vi "Configure Multi Eval Meas Trigger.vi"(0 "VISA resource name":refnum<visa-resource-name>, 1 "Trigger Threshold (-20.0)":dbl=-20.0 format="%^.3e", 2 "Minimum Trigger Gap (500e-6)":dbl=0.0005 format="%^.3e", 5 "Instance (1)":T1=1, 7 "Trigger Source (\"IF Power\")":string="IF Power", 9 "Trigger Slope (Rising)":i32(ring) items=["Rising", "Falling"], 11 "error in (no error)":errorcluster, 12 "Trigger Delay (0)":dbl format="%^.3e", 13 "Sync Mode (Normal)":i32(ring) items=["Normal", "Enhanced"]) -> (4 "VISA resource name out":refnum<visa-resource-name>, 15 "error out":errorcluster)   [LabVIEW 2020, in "Rohde&Schwarz CMWXP NR FR1 Measurement.lvlib"]
doc: "Configures multi evaluation measurement trigger subsystem.\n\nAttributes:\nRSCMWXPNRFR1M_ATTR_MULTI_EVAL_MEAS_TRIGGER_SOURCE\nRSCMWXPNRFR1M_ATTR_MULTI_EVAL_MEAS_TRIGGER_SLOPE\nRSCMWXPNRFR1M_ATTR_MULTI_EVAL_MEAS_TRIGGER_THRESHOLD\nRSCMWXPNRFR1M_ATTR_MULTI_EVAL_MEAS_TRIGGER_DELAY\nRSCMWXPNRFR1M_ATTR_MULTI_EVAL_MEAS_MINIMUM_TRIGGER_GAP\nRSCMWXPNRFR1M_ATTR_MULTI_EVAL_MEAS_TRIGGER_SYNC_MODE\n\nRemote-control commands:\nTRIGger:NRSub:MEAS<i>:MEValuation:SOURce\nTRIGger:NRSub:MEAS<i>:MEValuation:SLOPe\nTRIGger:NRSub:MEAS<i>:MEValuation:THReshold\nTRIGger:NRSub:MEAS<i>:MEValuation:DELay\nTRIGger:NRSub:MEAS<i>:MEValuation:MGAP\nTRIGger:NRSub:MEAS<i>:MEValuation:SMODe"
uses:
  <instrlib>/Rohde&Schwarz CMWXP NR FR1 Measurement/Rohde&Schwarz CMWXP NR FR1 Measurement.lvlib
  <instrlib>/Rohde&Schwarz CMWXP NR FR1 Measurement/Private/_Instance.ctl
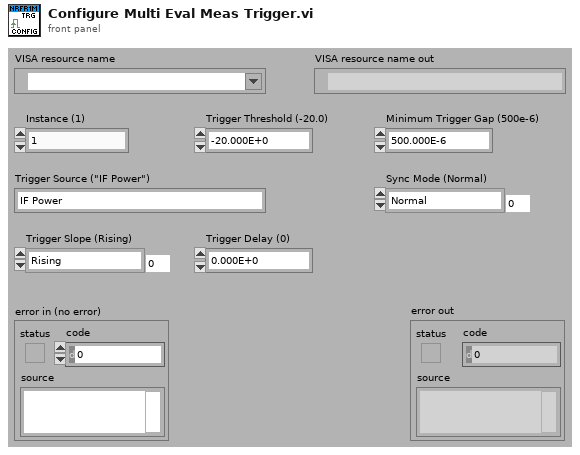
[diagram p1: front panel]
types:
  T1 = typedef "Rohde&Schwarz CMWXP NR FR1 Measurement.lvlib/_Instance.ctl" = i32
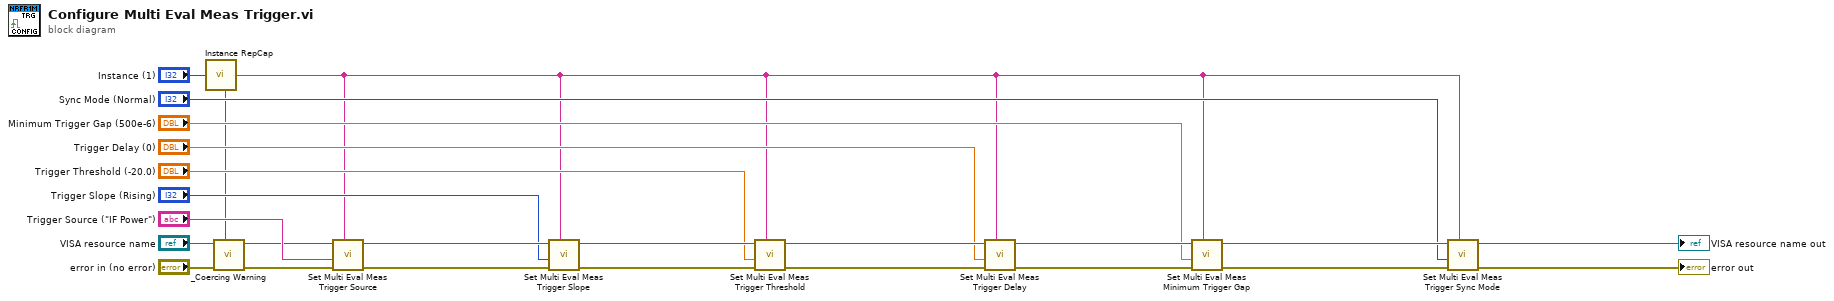
[diagram p0: block diagram]
diagram:
  n1 = call <instrlib>:"Instance RepCap.vi"("Instance In"="Instance (1)") -> ("In Range?"=w1:bool, "RepCap Identifier Out"=w6:string)  [unwired: 1 in]
  n2 = call <instrlib>:"_Coercing Warning.vi"("In Range?"=w1, "error in (no error)"="error in (no error)", "VISA resource name"="VISA resource name") -> ("error out"=w3:errorcluster, "VISA resource name out"=w2:refnum<visa-resource-name>)  [unwired: 7 in]
  n3 = call "Set Multi Eval Meas Trigger Source"("Repeated Capabilities"=w6, "error in (no error)"=w3, "Multi Eval Meas Trigger Source ()"="Trigger Source (\"IF Power\")", "instrument handle"=w2) -> ("error out"=w23:errorcluster, "instrument handle out"=w24:refnum<visa-resource-name>)  [unwired: 6 in]
  n4 = call "Set Multi Eval Meas Trigger Slope"("Repeated Capabilities"=w6, "error in (no error)"=w23, "Multi Eval Meas Trigger Slope (0 - Rising)"="Trigger Slope (Rising)", "instrument handle"=w24) -> ("error out"=w20:errorcluster, "instrument handle out"=w21:refnum<visa-resource-name>)  [unwired: 6 in]
  n5 = call "Set Multi Eval Meas Trigger Threshold"("Repeated Capabilities"=w6, "error in (no error)"=w20, "Multi Eval Meas Trigger Threshold (0.0)"="Trigger Threshold (-20.0)", "instrument handle"=w21) -> ("error out"=w17:errorcluster, "instrument handle out"=w18:refnum<visa-resource-name>)  [unwired: 6 in]
  n6 = call "Set Multi Eval Meas Trigger Delay"("Repeated Capabilities"=w6, "error in (no error)"=w17, "Multi Eval Meas Trigger Delay (0.0)"="Trigger Delay (0)", "instrument handle"=w18) -> ("error out"=w14:errorcluster, "instrument handle out"=w15:refnum<visa-resource-name>)  [unwired: 6 in]
  n7 = call "Set Multi Eval Meas Minimum Trigger Gap"("Repeated Capabilities"=w6, "error in (no error)"=w14, "Multi Eval Meas Minimum Trigger Gap (0.0)"="Minimum Trigger Gap (500e-6)", "instrument handle"=w15) -> ("error out"=w9:errorcluster, "instrument handle out"=w10:refnum<visa-resource-name>)  [unwired: 6 in]
  n8 = call "Set Multi Eval Meas Trigger Sync Mode"("Repeated Capabilities"=w6, "error in (no error)"=w9, "Multi Eval Meas Trigger Sync Mode (0 - Normal)"="Sync Mode (Normal)", "instrument handle"=w10) -> ("error out"=→"error out":errorcluster, "instrument handle out"=→"VISA resource name out":refnum<visa-resource-name>)  [unwired: 6 in]
